vi "Slow.vi"(9 "BackIn":dbl, 10 "RightIn":dbl, 11 "LeftIn":dbl) -> (1 "BackOut":dbl, 2 "RightOut":dbl, 3 "LeftOut":dbl)   [LabVIEW 2020]
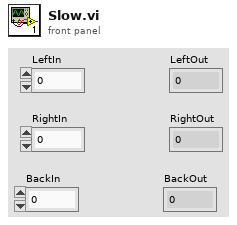
[diagram p1: front panel]
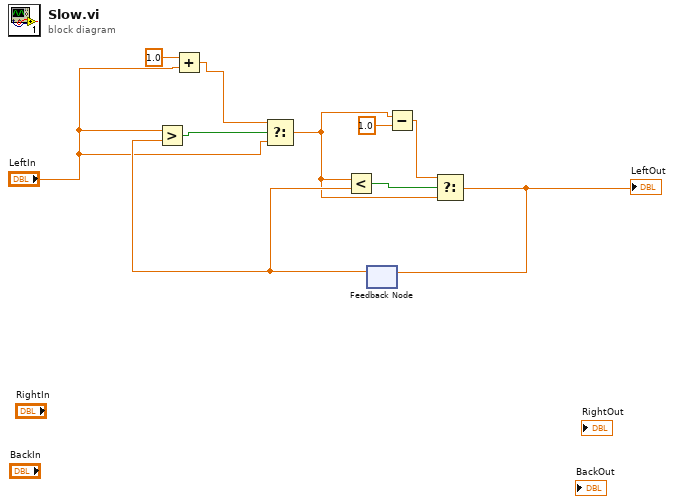
[diagram p0: block diagram]
diagram:
  n1 = Add(x=1.0, y="LeftIn") -> (x+y=w4:dbl)
  n2 = feedback #1() -> (w3:dbl)  [unwired: 1 in]
  n3 = Greater?(x="LeftIn", y=w3) -> (0:w10:bool)
  n4 = Select(t=w4, s=w10, f="LeftIn") -> (s? t:f=w2:dbl)
  n5 = Less?(x=w2, y=w3) -> (x < y?=w9:bool)
  n6 = Subtract(x=w2, y=1.0) -> (x-y=w5:dbl)
  n7 = Select(t=w5, s=w9, f=w2) -> (s? t:f=w8:dbl)
  "LeftOut" <- w8
  n8 = feedback-in #1(w8) -> ()
